vi "CC Focus Send Move Status.vi"(5 "data q":refnum<queue>, 7 "Names":string[](array[string]), 8 "error in (no error)":errorcluster, 10 "Moving":bool, 11 "motor":i32) -> (0 "error out":errorcluster)   [LabVIEW 2024]
uses:
  Subsystems/SS cluster Data Queue type.ctl
  hk-channel-class/hk-channel-class/HK Item/HK Channel cluster Telemetry Data.ctl
  hk-channel-class/hk-channel-class/HK Item/HK Channel enum Data Type.ctl
  hk-channel-class/hk-channel-class/HK Item/HK Item.lvclass
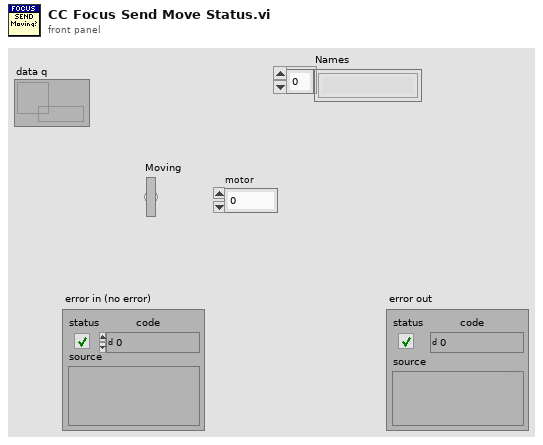
[diagram p1: front panel]
types:
  T1 = typedef "SS cluster Data Queue type.ctl" = cluster{"Source":string, "Type":string, "Data":variant}
  T2 = typedef "HK Item.lvclass/HK Channel enum Data Type.ctl" = enum16{"Floating Point", "Integer", "Enum", "String", "Waveform", "File"}
  T3 = typedef "HK Item.lvclass/HK Channel cluster Telemetry Data.ctl" = cluster{"Ch Names":string[], "Ch Values":dbl[], "Timestamp":timestamp, "Data Type":T2}
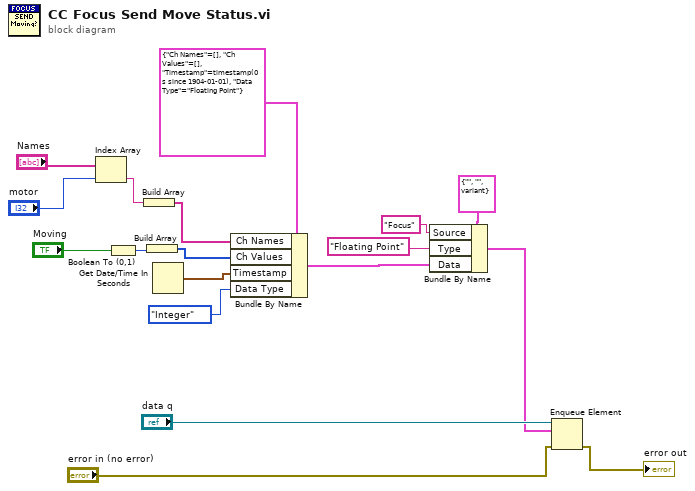
[diagram p0: block diagram]
diagram:
  n1 = Index Array(array="Names", index="motor") -> (element=w10:string)
  n2 = Boolean To (0,1)(Boolean="Moving") -> (0, 1=w14:i16)
  n3 = Build Array(w10) -> (w9:string[])
  n4 = Build Array(w14) -> (w13:i16[])
  n5 = Get Date/Time In Seconds() -> (seconds since 1Jan1904=w16:timestamp)
  n6 = Bundle By Name(cluster=T3 {"Ch Names"=[], "Ch Values"=[], "Timestamp"=timestamp(0 s since 1904-01-01), "Data Type"=enum."Floating Point"}, "Ch Names"=w9, "Ch Values"=w13, "Timestamp"=w16, "Data Type"=HK_Channel_enum_Data_Type."Integer") -> (w5:T3)
  n7 = Bundle By Name(cluster=T1 {"Source"="", "Type"="", "Data"=variant} ("element"), "Source"="Focus", "Type"="Floating Point" ("Data Type"), "Data"=w5) -> (w3:T1)
  n8 = Enqueue Element(queue="data q", element=w3, error in (no error)="error in (no error)") -> (error out=→"error out":errorcluster)  [unwired: 1 in, 2 out]
